vi "ScadeSend.vi"(11 "长度":i32=1 min=1 max=2) -> (3 "String":string)   [LabVIEW 2015]
uses:
  Global control/global-1.vi
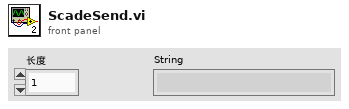
[diagram p1: front panel]
types:
  T1 = cluster{"60":bool, "70":bool, "2120":bool, "212":bool, "2121":bool, "2124":bool, "214":bool, "2140":bool, "2141":bool, "90":bool, "2110":bool, "211":bool, "2111":bool, "2113":bool, "备用1":bool, "备用2":bool}
  T2 = cluster{"225":bool, "201":bool, "202":bool, "226":bool, "236":bool, "236-7":bool, "237":bool, "237-7":bool, "231":bool, "231-7":bool, "245":bool, "2451":bool, "241":bool, "241-7":bool, "备用1":bool, "备用2":bool}
  T3 = cluster{"65":bool, "75":bool, "401":bool, "402":bool, "445":bool, "404":bool, "213":bool, "2130":bool, "2131":bool, "405":bool, "406":bool, "407":bool, "备用1":bool, "备用2":bool, "备用3":bool, "备用4":bool}
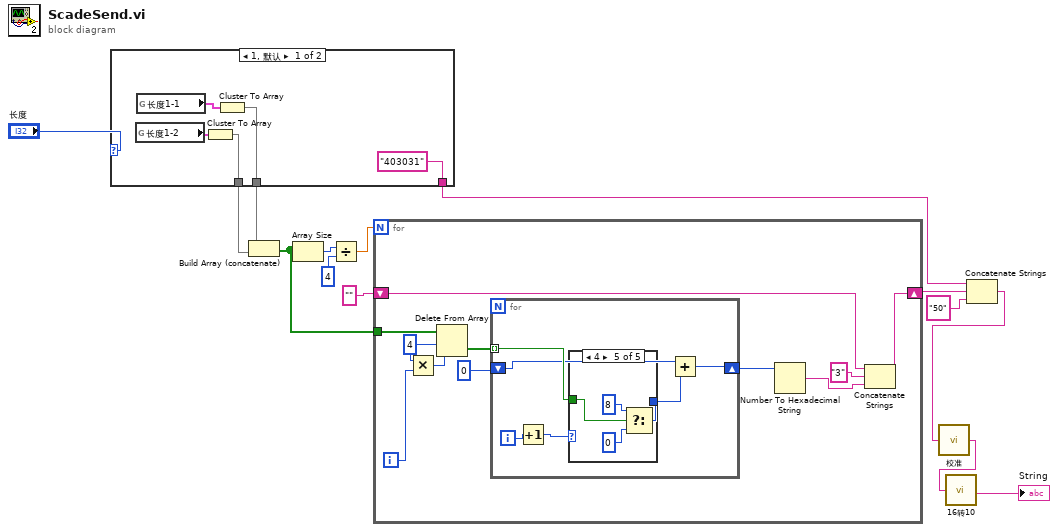
[diagram p0: block diagram]
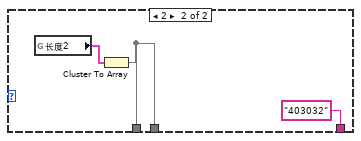
[diagram p2: hidden frame]
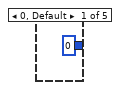
[diagram p3: hidden frame]
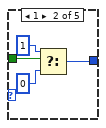
[diagram p4: hidden frame]
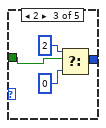
[diagram p5: hidden frame]
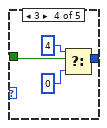
[diagram p6: hidden frame]
diagram:
  n1 = case shown="1, 默认" "长度" {
    tunnel: ["403031" ("字符串") "403032" ("字符串")] -> w9
    tunnel: [w17 w20] -> w3
    tunnel: [w16 w20] -> w2
    frame 1, Default {
      n2 = global read "global-1.vi" "长度1-2"() -> (w15:T1)
      n3 = global read "global-1.vi" "长度1-1"() -> (w18:T2)
      n4 = Cluster To Array(cluster=w15) -> (array=w16:bool[])
      n5 = Cluster To Array(cluster=w18) -> (array=w17:bool[])
    }
    frame 2 {
      n6 = global read "global-1.vi" "长度2"() -> (w21:T3)
      n7 = Cluster To Array(cluster=w21) -> (array=w20:bool[])
    }
  }
  n8 = Build Array (concatenate)(w3, w2) -> (w7:bool[])
  n9 = Array Size(array=w7) -> (size(s)=w4:i32)
  n10 = Divide(x=w4, y=4) -> (x/y=w6:dbl)
  n11 = for {
    N: w6 -> [_]
    tunnel: w7 -> [w33]
    shift-right: [w23] -> w10
    shift-left: "" ("字符串") -> [w24]
    i -> [w29]
    w31 = 4 ("长度")
    n12 = Multiply(x=w31, y=w29) -> (x*y=w32:i32)
    n13 = Delete From Array(array=w33, length=w31, index=w32) -> (deleted portion=w30:bool[])  [unwired: 1 out]
    n14 = for {
      tunnel: w30 -> [w37] mode=indexing
      shift-right: [w34] -> w27
      shift-left: 0 ("长度") -> [w36]
      i -> [w38]
      n15 = Increment(x=w38) -> (x+1=w39:i32)
      n16 = case shown="4" w39 {
        tunnel: w37 -> [_ w44 w46 w50 w54]
        tunnel: [0 ("长度") w41 w45 w49 w53] -> w35
        frame 0, Default {
        }
        frame 1 {
          n17 = Select(t=1 ("长度"), s=w44, f=0 ("长度")) -> (s? t:f=w41:i32)
        }
        frame 2 {
          n18 = Select(t=2 ("长度"), s=w46, f=0 ("长度")) -> (s? t:f=w45:i32)
        }
        frame 3 {
          n19 = Select(t=4 ("长度"), s=w50, f=0 ("长度")) -> (s? t:f=w49:i32)
        }
        frame 4 {
          n20 = Select(t=8 ("长度"), s=w54, f=0 ("长度")) -> (s? t:f=w53:i32)
        }
      }
      n21 = Add(x=w36, y=w35) -> (x+y=w34:i32)
    }
    n22 = Number To Hexadecimal String(2:w27) -> (0:w26:string)  [unwired: 1 in]
    n23 = Concatenate Strings(w24, "3" ("字符串"), w26) -> (w23:string)
  }
  n24 = Concatenate Strings(w9, w10, "50" ("字符串")) -> (w12:string)
  n25 = call "校准.vi"("字符串"=w12) -> ("连接的字符串"=w1:string)
  n26 = call "16转10.vi"("字符串"=w1) -> ("字符串 2"=→"String":string)
